vi "Do.vi"(8 "error in (no error)":errorcluster, 10 "Actor in":refnum<class "Actor.lvclass">, 11 "DNL_Message Template":refnum<class "Sequence State Msg.lvclass">) -> (0 "error out":errorcluster, 2 "Actor out":refnum<class "Actor.lvclass">)   [LabVIEW 2014, in "HIJ Vision Camera App Dialog.lvlib" / "Sequence State Msg.lvclass"]
doc: "This VI delivers the message to the actor by calling the appropriate method(s) on the actor."
uses:
  Sequence State Msg.lvclass
  <vilib>/ActorFramework/Actor/Actor.lvclass
  HIJ Vision Camera App Dialog/HIJ Vision Camera App Dialog.lvclass
  HIJ Vision Camera App/HIJ Vision Camera App Messages/Sequence State Msg/Sequence State Msg.lvclass/Sequence State Msg.ctl
  HIJ Vision Camera App/HIJ Vision Camera App Messages/Sequence State Msg/Read Current Nr_.vi
  HIJ Vision Camera App/HIJ Vision Camera App Messages/Sequence State Msg/Read Ready_.vi
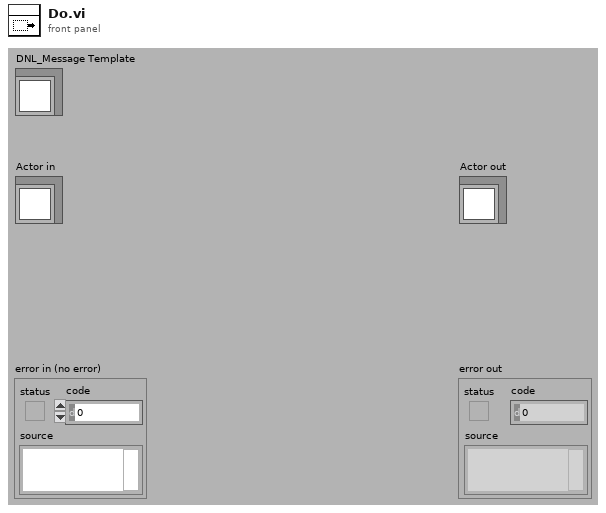
[diagram p1: front panel]
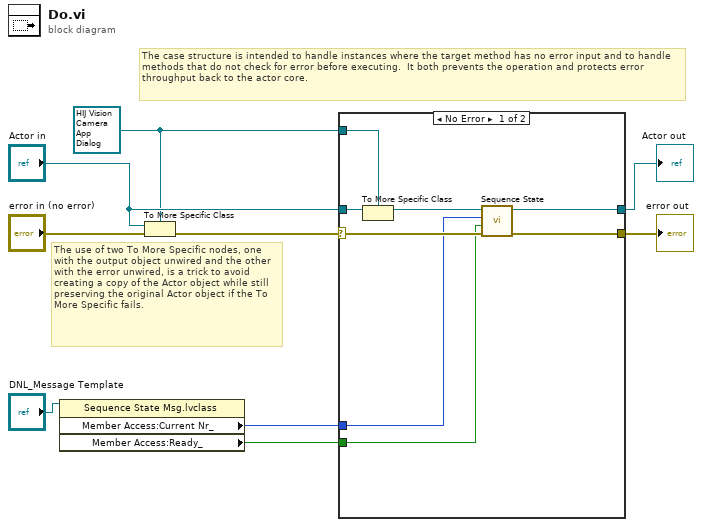
[diagram p0: block diagram]
diagram:
  w4 = refnum<class "HIJ Vision Camera App Dialog.lvclass"> refnum ("Actor in")
  # "The use of two To More Specific nodes, one with the output object unwired and the other with the error unwired, is a trick to avoid creating a copy of the Actor object while still preserving the original Actor object if the To More Specific fails."
  # "The case structure is intended to handle instances where the target method has no error input and to handle methods that do not check for error before executing.  It both prevents the operation and protects error throughput back to the actor core."
  n1 = property class="Sequence State Msg.lvclass"(reference="DNL_Message Template") -> ("Member Access:Current Nr_"=w2:u16, "Member Access:Ready_"=w1:bool)  [unwired: 1 in, 2 out]
  n2 = To More Specific Class(target class=w4, reference="Actor in", error in="error in (no error)") -> (error out=w8:errorcluster)  [unwired: 1 out]
  n3 = case shown="No Error" w8 {
    selector: w8 -> [w15 w19]
    tunnel: [w17 w19] -> w7
    tunnel: [w16 w18] -> w6
    tunnel: "Actor in" -> [w14 w18]
    tunnel: w4 -> [w13 _]
    tunnel: w2 -> [w11 _]
    tunnel: w1 -> [w10 _]
    frame No Error {
      n4 = To More Specific Class(target class=w13, reference=w14) -> (specific class reference=w12:refnum<class "HIJ Vision Camera App Dialog.lvclass">)  [unwired: 1 in, 1 out]
      n5 = call "Sequence State.vi"("error in (no error)"=w15, "Ready?"=w10, "Current Nr."=w11, "HIJ Vision Camera App Dialog in"=w12) -> ("error out"=w17:errorcluster, "HIJ Vision Camera App Dialog out"=w16:refnum<class "HIJ Vision Camera App Dialog.lvclass">)  [unwired: 6 in]
    }
    frame Error {
      # "If type check fails, pass the original object out again."
    }
  }
  "error out" <- w7
  "Actor out" <- w6
